vi "testt.vi"() -> ()   [LabVIEW 2023]
uses:
  <vilib>/Analysis/Matrix/Datatypes/RealMatrix.ctl
  <vilib>/Analysis/baseanly.llb/Real A x B.vi
  <vilib>/Utility/file.llb/Read Delimited Spreadsheet (DBL).vi
  <vilib>/Analysis/Matrix/Numeric/Add/Add - RM,RM.vi
  <vilib>/Analysis/NI_AALBase.lvlib
  <vilib>/Analysis/Matrix/NI_Matrix.lvlib
panel:
  out "Guess":i32[](array[numeric])
  out "Y":T1
  out "W2":T1
  out "Z1":T1
  out "W1":T1
  out "21":i32[](array[numeric])
  out "21 Z":dbl[][](array[numeric])
  out "B1":i32[](array[numeric])
  out "B2":i32[](array[numeric])
  out "A1":i32[](array[numeric])
  out "A2":i32[](array[numeric])
  out "B1":dbl[][](array[numeric])
  out "B2":dbl[][](array[numeric])
  out "A1":dbl[][](array[numeric])
  out "A2":dbl[][](array[numeric])
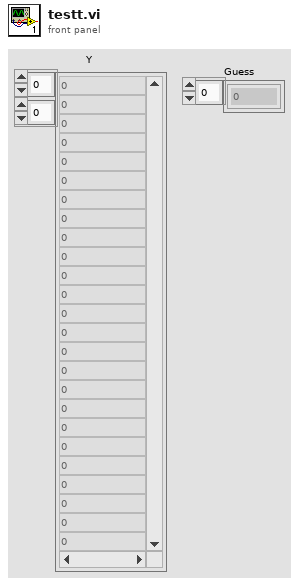
[diagram p1: front panel]
types:
  T1 = typedef "NI_Matrix.lvlib/RealMatrix.ctl" = dbl[][]
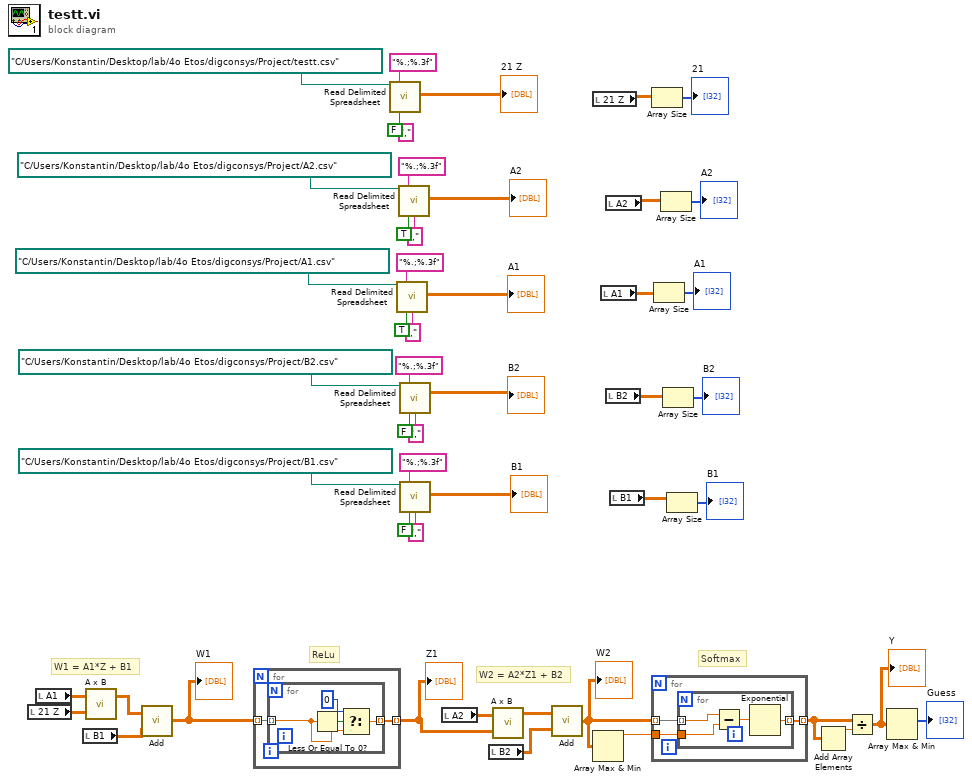
[diagram p0: block diagram]
diagram:
  (unwired) "," ("delimiter (\\t)")
  # "Softmax"
  # "W2 = A2*Z1 + B2"
  # "W1 = A1*Z + B1"
  # "ReLu"
  n1 = local read "21 Z"() -> (w16:dbl[][])
  n2 = local read "A1"() -> (w17:dbl[][])
  n3 = local read "B1"() -> (w14:dbl[][])
  n4 = call-poly <vilib>:"A x B.vi"("B"=w16, "A"=w17) -> ("A x B"=w15:T1)  [unwired: 1 out]
  n5 = call-poly <vilib>:"Add.vi"("Real Matrix B"=w14, "Real Matrix A"=w15) -> ("A + B"=w13:T1)
  "W1" <- w13
  n6 = for {
    tunnel: w13 -> [w51] mode=indexing
    tunnel: [w50] -> w9 mode=indexing
    n7 = for {
      tunnel: w51 -> [w54] mode=indexing
      tunnel: [w52] -> w50 mode=indexing
      n8 = Less Or Equal To 0?(x=w54) -> (x <= 0?=w55:bool)
      n9 = Select(t=0, s=w55, f=w54) -> (s? t:f=w52:dbl)
    }
  }
  "Z1" <- w9
  n10 = call-poly <vilib>:"Read Delimited Spreadsheet.vi"("file path (dialog if empty)"=path "C:/Users/Konstantin/Desktop/lab/4o Etos/digconsys/Project/testt.csv", "format (%.3f)"="%.;%.3f", "transpose? (F)"=FALSE) -> ("all rows"=→"21 Z":dbl[][])  [unwired: 7 in, 5 out]
  n11 = call-poly <vilib>:"Read Delimited Spreadsheet.vi"("file path (dialog if empty)"=path "C:/Users/Konstantin/Desktop/lab/4o Etos/digconsys/Project/A1.csv", "format (%.3f)"="%.;%.3f", "transpose? (F)"=TRUE, "delimiter (\\t)"="," ("delimiter (\\t)")) -> ("all rows"=→"A1":dbl[][])  [unwired: 6 in, 5 out]
  n12 = call-poly <vilib>:"Read Delimited Spreadsheet.vi"("file path (dialog if empty)"=path "C:/Users/Konstantin/Desktop/lab/4o Etos/digconsys/Project/A2.csv", "format (%.3f)"="%.;%.3f", "transpose? (F)"=TRUE, "delimiter (\\t)"="," ("delimiter (\\t)")) -> ("all rows"=→"A2":dbl[][])  [unwired: 6 in, 5 out]
  n13 = call-poly <vilib>:"Read Delimited Spreadsheet.vi"("file path (dialog if empty)"=path "C:/Users/Konstantin/Desktop/lab/4o Etos/digconsys/Project/B2.csv", "format (%.3f)"="%.;%.3f", "transpose? (F)"=FALSE, "delimiter (\\t)"="," ("delimiter (\\t)")) -> ("all rows"=→"B2":dbl[][])  [unwired: 6 in, 5 out]
  n14 = call-poly <vilib>:"Read Delimited Spreadsheet.vi"("file path (dialog if empty)"=path "C:/Users/Konstantin/Desktop/lab/4o Etos/digconsys/Project/B1.csv", "format (%.3f)"="%.;%.3f", "transpose? (F)"=FALSE, "delimiter (\\t)"="," ("delimiter (\\t)")) -> ("all rows"=→"B1":dbl[][])  [unwired: 6 in, 5 out]
  n15 = local read "A2"() -> (w10:dbl[][])
  n16 = local read "B2"() -> (w7:dbl[][])
  n17 = call-poly <vilib>:"A x B.vi"("B"=w9, "A"=w10) -> ("A x B"=w8:T1)  [unwired: 1 out]
  n18 = call-poly <vilib>:"Add.vi"("Real Matrix B"=w7, "Real Matrix A"=w8) -> ("A + B"=w6:T1)
  "W2" <- w6
  n19 = local read "21 Z"() -> (w19:dbl[][])
  n20 = Array Max & Min(array=w6) -> (max value=w5:dbl)  [unwired: 3 out]
  n21 = local read "A1"() -> (w26:dbl[][])
  n22 = local read "A2"() -> (w31:dbl[][])
  n23 = local read "B2"() -> (w25:dbl[][])
  n24 = local read "B1"() -> (w24:dbl[][])
  n25 = Array Size(array=w19) -> (size(s)=→"21":i32[])
  n26 = for {
    tunnel: w6 -> [w58] mode=indexing
    tunnel: w5 -> [w57]
    tunnel: [w56] -> w3 mode=indexing
    n27 = for {
      tunnel: w58 -> [w62] mode=indexing
      tunnel: w57 -> [w61]
      tunnel: [w59] -> w56 mode=indexing
      n28 = Subtract(x=w62, y=w61) -> (x-y=w60:dbl)
      n29 = Exponential(1:w60) -> (0:w59:dbl)
    }
  }
  n30 = Array Size(array=w26) -> (size(s)=→"A1":i32[])
  n31 = Array Size(array=w31) -> (size(s)=→"A2":i32[])
  n32 = Array Size(array=w25) -> (size(s)=→"B2":i32[])
  n33 = Array Size(array=w24) -> (size(s)=→"B1":i32[])
  n34 = Add Array Elements(numeric array=w3) -> (sum=w4:dbl)
  n35 = Divide(x=w3, y=w4) -> (x/y=w2:dbl[][])
  "Y" <- w2
  n36 = Array Max & Min(array=w2) -> (max index (indices)=→"Guess":i32[])  [unwired: 3 out]
